vi "construct hex string.vi"() -> ()   [LabVIEW 2016]
panel:
  out "after match out 2":string
  out "after match out":string
  out "error out":errorcluster
  out "status word":u32 format="0x%02x"
  out "status string out":string
  out "Address":u32 format="0x%02x"
  out "Address":string
  out "after match":string
  in  "String":string
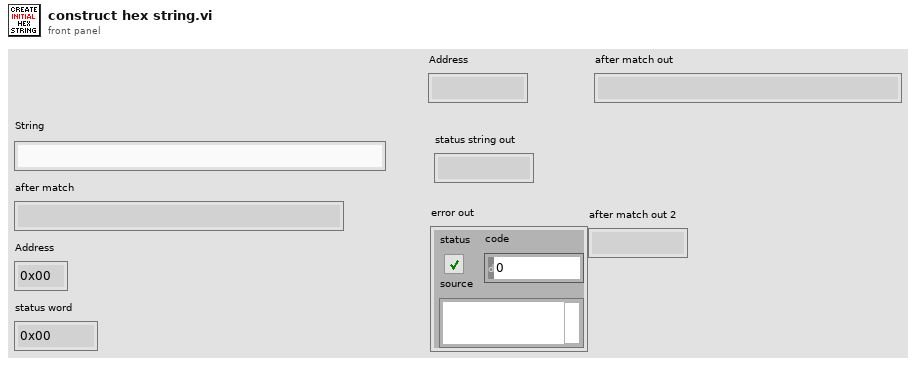
[diagram p1: front panel]
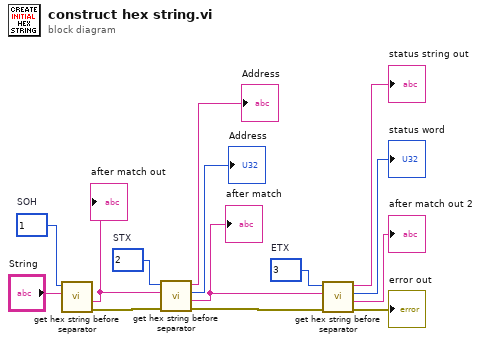
[diagram p0: block diagram]
diagram:
  w6 = 3  # ETX
  w14 = 2  # STX
  w11 = 1  # SOH
  n1 = call "get hex string before separator.vi"("String In"="String", "Separator In"=w11) -> ("error out"=w9:errorcluster, "after match out"=w8:string)  [unwired: 6 in, 2 out]
  "after match out" <- w8
  n2 = call "get hex string before separator.vi"("error in (no error)"=w9, "String In"=w8, "Separator In"=w14) -> ("error out"=w5:errorcluster, "after match out"=w7:string, "hexadecimal out"=→"Address":u32, "hexadecimal string out"=→"Address":string)  [unwired: 5 in]
  "after match" <- w7
  n3 = call "get hex string before separator.vi"("error in (no error)"=w5, "String In"=w7, "Separator In"=w6) -> ("error out"=→"error out":errorcluster, "after match out"=→"after match out 2":string, "hexadecimal out"=→"status word":u32, "hexadecimal string out"=→"status string out":string)  [unwired: 5 in]
